vi "RF-Power-On-OFF.vi"(8 "error in (no error)":errorcluster, 9 "RF Power State (T: On)":bool, 11 "C4209 PNA":refnum<class "C4209 PNA.lvclass">) -> (0 "error out":errorcluster, 3 "C4209 PNA out":refnum<class "C4209 PNA.lvclass">)   [LabVIEW 2017, in "C4209 PNA.lvclass"]
uses:
  C4209 PNA.lvclass
  C4209 PNA.lvclass/C4209 PNA.ctl
  <instrlib>/CMT S2 Series VNA/CMT S2 Series VNA.lvlib
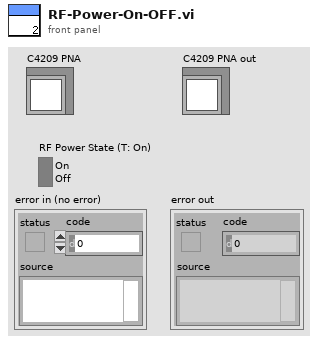
[diagram p1: front panel]
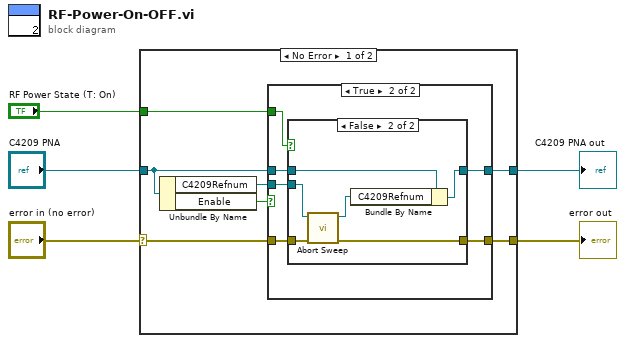
[diagram p0: block diagram]
diagram:
  n1 = case shown="No Error" "error in (no error)" {
    selector: "error in (no error)" -> [w10 w30]
    tunnel: [w9 w30] -> w4
    tunnel: [w11 w29] -> w2
    tunnel: "C4209 PNA" -> [w12 w29]
    tunnel: "RF Power State (T: On)" -> [w7 _]
    frame No Error {
      n2 = Unbundle By Name(w12) -> ("C4209Refnum"=w8:refnum<k7>, "Enable"=w6:bool)
      n3 = case shown="True" w6 {
        tunnel: w12 -> [w14 w20]
        tunnel: [w14 w19] -> w11
        tunnel: w10 -> [w13 w18]
        tunnel: [w13 w17] -> w9
        tunnel: w8 -> [_ w16]
        tunnel: w7 -> [_ w15]
        frame False {
        }
        frame True {
          n4 = case shown="False" w15 {
            tunnel: w20 -> [w22 w27]
            tunnel: [w22 w28] -> w19
            tunnel: w18 -> [w21 w24]
            tunnel: [w21 w23] -> w17
            tunnel: w16 -> [_ w26]
            frame True {
            }
            frame False {
              n5 = call <instrlib>:"Abort Sweep.vi"("error in (no error)"=w24, "Reference in"=w26) -> ("error out"=w23:errorcluster, "Reference out"=w25:refnum<k7>)  [unwired: 8 in]
              n6 = Bundle By Name(cluster=w27, "C4209Refnum"=w25) -> (w28:refnum<class "C4209 PNA.lvclass">)
            }
          }
        }
      }
    }
    frame Error {
    }
  }
  "error out" <- w4
  "C4209 PNA out" <- w2
